vi "process.vi"(8 "error in":errorcluster, 9 "result allocation":T1, 10 "parameters":T1, 11 "GPIC ScaleAndLimit runtime in":refnum<class "GPIC ScaleAndLimit runtime.lvclass">) -> (0 "error out":errorcluster, 1 "results":T1, 2 "parameter allocation":T1, 3 "GPIC ScaleAndLimit runtime out":refnum<class "GPIC ScaleAndLimit runtime.lvclass">)   [LabVIEW 2015, in "GPIC ScaleAndLimit runtime.lvclass"]
doc: "Provides an interface for information processing by a module at runtime. While this interface performs no operations, a child should provide an override which may process data in any manner necessary."
uses:
  GPIC ScaleAndLimit runtime.lvclass
  <vilib>/NI/Tag Bus/table/data table.ctl
  GPIC ScaleAndLimit runtime.lvclass/GPIC ScaleAndLimit runtime.ctl
  <vilib>/NI/Tag Bus/table/data table.lvlib
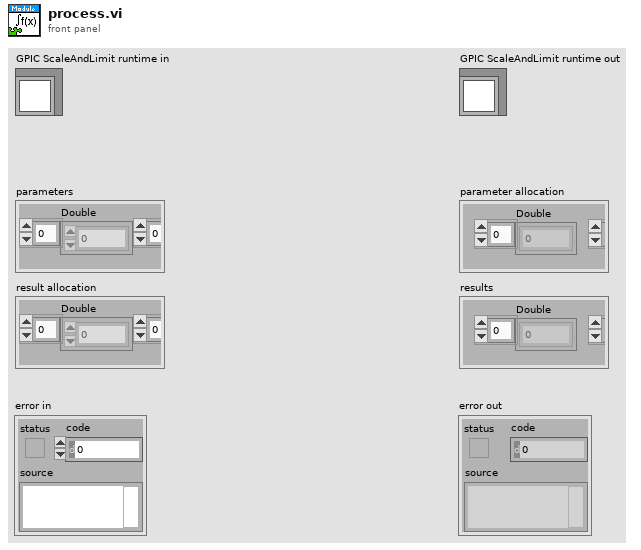
[diagram p1: front panel]
types:
  T1 = typedef "tag bus.lvlib/data table.lvlib/data table.ctl" = cluster{"Double":dbl[], "Single":sgl[], "I64":i64[], "I32":i32[], "I16":i16[], "I8":i8[], "U64":u64[], "U32":u32[], "U16":u16[], "U8":u8[], "Boolean":bool[], "String":string[], "Array of Double":cluster{"DBL Array":dbl[]}[], "Array of Single":cluster{"SGL Array":sgl[]}[], "Array of I64":cluster{"I64 Array":i64[]}[], "Array of I32":cluster{"I32 Array":i32[]}[], "Array of I16":cluster{"I16 Array":i16[]}[], "Array of I8":cluster{"I8 Array":i8[]}[], "Array of U64":cluster{"U64 Array":u64[]}[], "Array of U32":cluster{"U32 Array":u32[]}[], "Array of U16":cluster{"U16 Array":u16[]}[], "Array of U8":cluster{"U8 Array":u8[]}[], "Array of Boolean":cluster{"Boolean Array":bool[]}[], "Array of String":cluster{"String Array":string[]}[]}
  T2 = typedef "GPIC ScaleAndLimit configuration.lvclass/parameter data indices.ctl" = cluster{"fmwk_placeholder":i32}
  T3 = typedef "GPIC ScaleAndLimit configuration.lvclass/result data indices.ctl" = cluster{"fmwk_placeholder":i32}
  T4 = typedef "GPIC ScaleAndLimit runtime.lvclass/parameter user data.ctl" = cluster{"fmwk_placeholder":i32}
  T5 = typedef "GPIC ScaleAndLimit runtime.lvclass/result user data.ctl" = cluster{"fmwk_placeholder":i32}
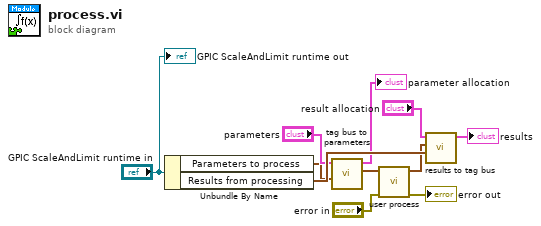
[diagram p0: block diagram]
diagram:
  n1 = Unbundle By Name("GPIC ScaleAndLimit runtime in") -> ("Parameters to process"=w3:T2, "Results from processing"=w6:T3)
  n2 = call "tag bus to parameters.vi"("indices"=w3, "tag bus in"="parameters") -> ("data cluster"=w2:T4, "tag bus out"=→"parameter allocation":T1)  [unwired: 8 in]
  n3 = call "user process.vi"("error in"="error in", "Parameters to process"=w2) -> ("error out"=→"error out":errorcluster, "Results from processing"=w1:T5)  [unwired: 8 in]
  n4 = call "results to tag bus.vi"("indices"=w6, "data cluster"=w1, "tag bus in"="result allocation") -> ("tag bus out"=→"results":T1)  [unwired: 8 in]
  "GPIC ScaleAndLimit runtime out" <- "GPIC ScaleAndLimit runtime in"
